vi "Static field instruction generator (SubVI).vi"(9 "Magnetic field strength z [µT]":dbl, 10 "Magnetic field strength y [µT]":dbl, 11 "Magnetic field strength x [µT]":dbl) -> (1 "Necessary current Y":dbl, 2 "Necessary current X":dbl, 3 "Necessary current Z":dbl, 4 "String":string)   [LabVIEW 2018]
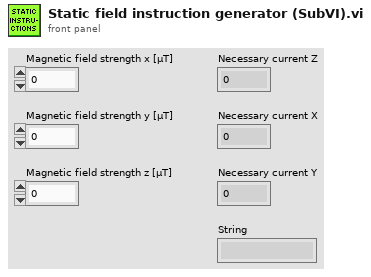
[diagram p1: front panel]
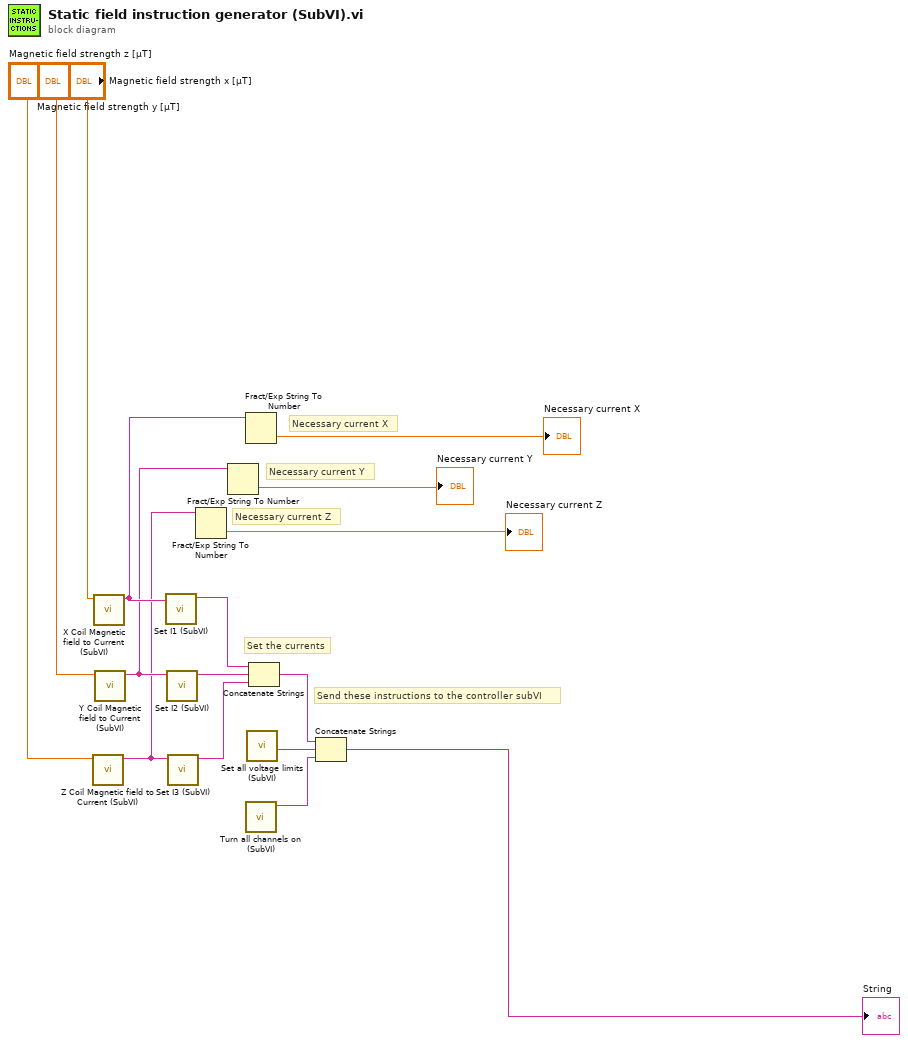
[diagram p0: block diagram]
diagram:
  # "Send these instructions to the controller subVI"
  # "Set the currents"
  # "Necessary current Z"
  # "Necessary current Y"
  # "Necessary current X"
  n1 = call "Z Coil Magnetic field to Current (SubVI).vi"("Magnetic field [µT]"="Magnetic field strength z [µT]") -> ("Current Z"=w1:string)  [unwired: 10 in]
  n2 = call "X Coil Magnetic field to Current (SubVI).vi"("Magnetic field [µT]"="Magnetic field strength x [µT]") -> ("Current X"=w3:string)  [unwired: 10 in]
  n3 = call "Y Coil Magnetic field to Current (SubVI).vi"("Magnetic field [µT]"="Magnetic field strength y [µT]") -> ("Current Y"=w2:string)  [unwired: 10 in]
  n4 = call "Set I1 (SubVI).vi"("Current X"=w3) -> ("String instruction"=w9:string)  [unwired: 10 in]
  n5 = call "Set I2 (SubVI).vi"("Current Y"=w2) -> ("String"=w8:string)  [unwired: 10 in]
  n6 = call "Set I3 (SubVI).vi"("Current Z"=w1) -> ("String"=w7:string)  [unwired: 10 in]
  n7 = Fract/Exp String To Number(string=w1) -> (number=→"Necessary current Z":dbl)  [unwired: 3 in, 1 out]
  n8 = Fract/Exp String To Number(string=w2) -> (number=→"Necessary current Y":dbl)  [unwired: 3 in, 1 out]
  n9 = Fract/Exp String To Number(string=w3) -> (number=→"Necessary current X":dbl)  [unwired: 3 in, 1 out]
  n10 = call "Turn all channels on (SubVI).vi"() -> ("String"=w4:string)  [unwired: 11 in]
  n11 = call "Set all voltage limits (SubVI).vi"() -> ("String"=w5:string)  [unwired: 11 in]
  n12 = Concatenate Strings(w9, w8, w7) -> (w6:string)
  n13 = Concatenate Strings(w6, w5, w4) -> (→"String":string)
